vi "GetProbePlanCoordinates.vi"(8 "Use index as X coord":bool=TRUE, 9 "Probe Card Channels":i32=1) -> (0 "file path":string="C:\\Users\\itk\\Documents\\itk-strip-sensor-qc\\ProbePlans\\190723_ATLAS18R0_layer5__ATLAS18R0_ACPads.txt", 2 "OK?":bool=TRUE, 3 "Array":T1(array[cluster])=[{"Region"="Segment\t0T", "ProbePoints"=[{"X"=1.0, "Y"=0.0, "Label"="Strip\t1", "Coord On/Off"=TRUE}, {"X"=2.0, "Y"=0.0, "Label"="Strip\t2", "Coord On/Off"=TRUE}, {"X"=3.0, "Y"=0.0, "Label"="Strip\t3", "Coord On/Off"=TRUE}, {"X"=4.0, "Y"=0.0, "Label"="Strip\t4", "Coord On/Off"=TRUE}, {"X"=5.0, "Y"=0.0, "Label"="Strip\t5", "Coord On/Off"=TRUE}, {"X"=6.0, "Y"=0.0, "Label"="Strip\t6", "Coord On/Off"=TRUE}, {"X"=7.0, "Y"=0.0, "Label"="Strip\t7", "Coord On/Off"=TRUE}, {"X"=8.0, "Y"=0.0, "Label"="Strip\t8", "Coord On/Off"=TRUE}, {"X"=9.0, "Y"=0.0, "Label"="Strip\t9", "Coord On/Off"=TRUE}, {"X"=10.0, "Y"=0.0, "Label"="Strip\t10", "Coord On/Off"=TRUE}, {"X"=11.0, "Y"=0.0, "Label"="Strip\t11", "Coord On/Off"=TRUE}, {"X"=12.0, "Y"=0.0, "Label"="Strip\t12", "Coord On/Off"=TRUE}, {"X"=13.0, "Y"=0.0, "Label"="Strip\t13", "Coord On/Off"=TRUE}, {"X"=14.0, "Y"=0.0, "Label"="Strip\t14", "Coord On/Off"=TRUE}, {"X"=15.0, "Y"=0.0, "Label"="Strip\t15", "Coord On/Off"=TRUE}, {"X"=16.0, "Y"=0.0, "Label"="Strip\t16", "Coord On/Off"=TRUE}, {"X"=17.0, "Y"=0.0, "Label"="Strip\t17", "Coord On/Off"=TRUE}, {"X"=18.0, "Y"=0.0, "Label"="Strip\t18", "Coord On/Off"=TRUE}, {"X"=19.0, "Y"=0.0, "Label"="Strip\t19", "Coord On/Off"=TRUE}, {"X"=20.0, "Y"=0.0, "Label"="Strip\t20", "Coord On/Off"=TRUE}, {"X"=21.0, "Y"=0.0, "Label"="Strip\t21", "Coord On/Off"=TRUE}, {"X"=22.0, "Y"=0.0, "Label"="Strip\t22", "Coord On/Off"=TRUE}, {"X"=23.0, "Y"=0.0, "Label"="Strip\t23", "Coord On/Off"=TRUE}, {"X"=24.0, "Y"=0.0, "Label"="Strip\t24", "Coord On/Off"=TRUE}, {"X"=25.0, "Y"=0.0, "Label"="Strip\t25", "Coord On/Off"=TRUE}, {"X"=26.0, "Y"=0.0, "Label"="Strip\t26", "Coord On/Off"=TRUE}, {"X"=27.0, "Y"=0.0, "Label"="Strip\t27", "Coord On/Off"=TRUE}, {"X"=28.0, "Y"=0.0, "Label"="Strip\t28", "Coord On/Off"=TRUE}, {"X"=29.0, "Y"=0.0, "Label"="Strip\t29", "Coord On/Off"=TRUE}, {"X"=30.0, "Y"=0.0, "Label"="Strip\t30", "Coord On/Off"=TRUE}, {"X"=31.0, "Y"=0.0, "Label"="Strip\t31", "Coord On/Off"=TRUE}, {"X"=32.0, "Y"=0.0, "Label"="Strip\t32", "Coord On/Off"=TRUE}, {"X"=33.0, "Y"=0.0, "Label"="Strip\t33", "Coord On/Off"=TRUE}, {"X"=34.0, "Y"=0.0, "Label"="Strip\t34", "Coord On/Off"=TRUE}, {"X"=35.0, "Y"=0.0, "Label"="Strip\t35", "Coord On/Off"=TRUE}, {"X"=36.0, "Y"=0.0, "Label"="Strip\t36", "Coord On/Off"=TRUE}, {"X"=37.0, "Y"=0.0, "Label"="Strip\t37", "Coord On/Off"=TRUE}, {"X"=38.0, "Y"=0.0, "Label"="Strip\t38", "Coord On/Off"=TRUE}, {"X"=39.0, "Y"=0.0, "Label"="Strip\t39", "Coord On/Off"=TRUE}, {"X"=40.0, "Y"=0.0, "Label"="Strip\t40", "Coord On/Off"=TRUE}, {"X"=41.0, "Y"=0.0, "Label"="Strip\t41", "Coord On/Off"=TRUE}, {"X"=42.0, "Y"=0.0, "Label"="Strip\t42", "Coord On/Off"=TRUE}, {"X"=43.0, "Y"=0.0, "Label"="Strip\t43", "Coord On/Off"=TRUE}, {"X"=44.0, "Y"=0.0, "Label"="Strip\t44", "Coord On/Off"=TRUE}, {"X"=45.0, "Y"=0.0, "Label"="Strip\t45", "Coord On/Off"=TRUE}, {"X"=46.0, "Y"=0.0, "Label"="Strip\t46", "Coord On/Off"=TRUE}, {"X"=47.0, "Y"=0.0, "Label"="Strip\t47", "Coord On/Off"=TRUE}, {"X"=48.0, "Y"=0.0, "Label"="Strip\t48", "Coord On/Off"=TRUE}, {"X"=49.0, "Y"=0.0, "Label"="Strip\t49", "Coord On/Off"=TRUE}, {"X"=50.0, "Y"=0.0, "Label"="Strip\t50", "Coord On/Off"=TRUE}, {"X"=51.0, "Y"=0.0, "Label"="Strip\t51", "Coord On/Off"=TRUE}, {"X"=52.0, "Y"=0.0, "Label"="Strip\t52", "Coord On/Off"=TRUE}, {"X"=53.0, "Y"=0.0, "Label"="Strip\t53", "Coord On/Off"=TRUE}, {"X"=54.0, "Y"=0.0, "Label"="Strip\t54", "Coord On/Off"=TRUE}, {"X"=55.0, "Y"=0.0, "Label"="Strip\t55", "Coord On/Off"=TRUE}, {"X"=56.0, "Y"=0.0, "Label"="Strip\t56", "Coord On/Off"=TRUE}, {"X"=57.0, "Y"=0.0, "Label"="Strip\t57", "Coord On/Off"=TRUE}, {"X"=58.0, "Y"=0.0, "Label"="Strip\t58", "Coord On/Off"=TRUE}, {"X"=59.0, "Y"=0.0, "Label"="Strip\t59", "Coord On/Off"=TRUE}, {"X"=60.0, "Y"=0.0, "Label"="Strip\t60", "Coord On/Off"=TRUE}, {"X"=61.0, "Y"=0.0, "Label"="Strip\t61", "Coord On/Off"=TRUE}, {"X"=62.0, "Y"=0.0, "Label"="Strip\t62", "Coord On/Off"=TRUE}, {"X"=63.0, "Y"=0.0, "Label"="Strip\t63", "Coord On/Off"=TRUE}, {"X"=64.0, "Y"=0.0, "Label"="Strip\t64", "Coord On/Off"=TRUE}, {"X"=65.0, "Y"=0.0, "Label"="Strip\t65", "Coord On/Off"=TRUE}, {"X"=66.0, "Y"=0.0, "Label"="Strip\t66", "Coord On/Off"=TRUE}, {"X"=67.0, "Y"=0.0, "Label"="Strip\t67", "Coord On/Off"=TRUE}, {"X"=68.0, "Y"=0.0, "Label"="Strip\t68", "Coord On/Off"=TRUE}, {"X"=69.0, "Y"=0.0, "Label"="Strip\t69", "Coord On/Off"=TRUE}, {"X"=70.0, "Y"=0.0, "Label"="Strip\t70", "Coord On/Off"=TRUE}, {"X"=71.0, "Y"=0.0, "Label"="Strip\t71", "Coord On/Off"=TRUE}, {"X"=72.0, "Y"=0.0, "Label"="Strip\t72", "Coord On/Off"=TRUE}, {"X"=73.0, "Y"=0.0, "Label"="Strip\t73", "Coord On/Off"=TRUE}, {"X"=74.0, "Y"=0.0, "Label"="Strip\t74", "Coord On/Off"=TRUE}, {"X"=75.0, "Y"=0.0, "Label"="Strip\t75", "Coord On/Off"=TRUE}, {"X"=76.0, "Y"=0.0, "Label"="Strip\t76", "Coord On/Off"=TRUE}, {"X"=77.0, "Y"=0.0, "Label"="Strip\t77", "Coord On/Off"=TRUE}, {"X"=78.0, "Y"=0.0, "Label"="Strip\t78", "Coord On/Off"=TRUE}, {"X"=79.0, "Y"=0.0, "Label"="Strip\t79", "Coord On/Off"=TRUE}, {"X"=80.0, "Y"=0.0, "Label"="Strip\t80", "Coord On/Off"=TRUE}, {"X"=81.0, "Y"=0.0, "Label"="Strip\t81", "Coord On/Off"=TRUE}, {"X"=82.0, "Y"=0.0, "Label"="Strip\t82", "Coord On/Off"=TRUE}, {"X"=83.0, "Y"=0.0, "Label"="Strip\t83", "Coord On/Off"=TRUE}, {"X"=84.0, "Y"=0.0, "Label"="Strip\t84", "Coord On/Off"=TRUE}, {"X"=85.0, "Y"=0.0, "Label"="Strip\t85", "Coord On/Off"=TRUE}, {"X"=86.0, "Y"=0.0, "Label"="Strip\t86", "Coord On/Off"=TRUE}, {"X"=87.0, "Y"=0.0, "Label"="Strip\t87", "Coord On/Off"=TRUE}, {"X"=88.0, "Y"=0.0, "Label"="Strip\t88", "Coord On/Off"=TRUE}, {"X"=89.0, "Y"=0.0, "Label"="Strip\t89", "Coord On/Off"=TRUE}, {"X"=90.0, "Y"=0.0, "Label"="Strip\t90", "Coord On/Off"=TRUE}, {"X"=91.0, "Y"=0.0, "Label"="Strip\t91", "Coord On/Off"=TRUE}, {"X"=92.0, "Y"=0.0, "Label"="Strip\t92", "Coord On/Off"=TRUE}, {"X"=93.0, "Y"=0.0, "Label"="Strip\t93", "Coord On/Off"=TRUE}, {"X"=94.0, "Y"=0.0, "Label"="Strip\t94", "Coord On/Off"=TRUE}, {"X"=95.0, "Y"=0.0, "Label"="Strip\t95", "Coord On/Off"=TRUE}, {"X"=96.0, "Y"=0.0, "Label"="Strip\t96", "Coord On/Off"=TRUE}, {"X"=97.0, "Y"=0.0, "Label"="Strip\t97", "Coord On/Off"=TRUE}, {"X"=98.0, "Y"=0.0, "Label"="Strip\t98", "Coord On/Off"=TRUE}, {"X"=99.0, "Y"=0.0, "Label"="Strip\t99", "Coord On/Off"=TRUE}, {"X"=100.0, "Y"=0.0, "Label"="Strip\t100", "Coord On/Off"=TRUE}, {"X"=101.0, "Y"=0.0, "Label"="Strip\t101", "Coord On/Off"=TRUE}, {"X"=102.0, "Y"=0.0, "Label"="Strip\t102", "Coord On/Off"=TRUE}, {"X"=103.0, "Y"=0.0, "Label"="Strip\t103", "Coord On/Off"=TRUE}, {"X"=104.0, "Y"=0.0, "Label"="Strip\t104", "Coord On/Off"=TRUE}, {"X"=105.0, "Y"=0.0, "Label"="Strip\t105", "Coord On/Off"=TRUE}, {"X"=106.0, "Y"=0.0, "Label"="Strip\t106", "Coord On/Off"=TRUE}, {"X"=107.0, "Y"=0.0, "Label"="Strip\t107", "Coord On/Off"=TRUE}, {"X"=108.0, "Y"=0.0, "Label"="Strip\t108", "Coord On/Off"=TRUE}, {"X"=109.0, "Y"=0.0, "Label"="Strip\t109", "Coord On/Off"=TRUE}, {"X"=110.0, "Y"=0.0, "Label"="Strip\t110", "Coord On/Off"=TRUE}, {"X"=111.0, "Y"=0.0, "Label"="Strip\t111", "Coord On/Off"=TRUE}, {"X"=112.0, "Y"=0.0, "Label"="Strip\t112", "Coord On/Off"=TRUE}, {"X"=113.0, "Y"=0.0, "Label"="Strip\t113", "Coord On/Off"=TRUE}, {"X"=114.0, "Y"=0.0, "Label"="Strip\t114", "Coord On/Off"=TRUE}, {"X"=115.0, "Y"=0.0, "Label"="Strip\t115", "Coord On/Off"=TRUE}, {"X"=116.0, "Y"=0.0, "Label"="Strip\t116", "Coord On/Off"=TRUE}, {"X"=117.0, "Y"=0.0, "Label"="Strip\t117", "Coord On/Off"=TRUE}, {"X"=118.0, "Y"=0.0, "Label"="Strip\t118", "Coord On/Off"=TRUE}, {"X"=119.0, "Y"=0.0, "Label"="Strip\t119", "Coord On/Off"=TRUE}, {"X"=120.0, "Y"=0.0, "Label"="Strip\t120", "Coord On/Off"=TRUE}, {"X"=121.0, "Y"=0.0, "Label"="Strip\t121", "Coord On/Off"=TRUE}, {"X"=122.0, "Y"=0.0, "Label"="Strip\t122", "Coord On/Off"=TRUE}, {"X"=123.0, "Y"=0.0, "Label"="Strip\t123", "Coord On/Off"=TRUE}, {"X"=124.0, "Y"=0.0, "Label"="Strip\t124", "Coord On/Off"=TRUE}, {"X"=125.0, "Y"=0.0, "Label"="Strip\t125", "Coord On/Off"=TRUE}, {"X"=126.0, "Y"=0.0, "Label"="Strip\t126", "Coord On/Off"=TRUE}, {"X"=127.0, "Y"=0.0, "Label"="Strip\t127", "Coord On/Off"=TRUE}, {"X"=128.0, "Y"=0.0, "Label"="Strip\t128", "Coord On/Off"=TRUE}, {"X"=129.0, "Y"=0.0, "Label"="Strip\t129", "Coord On/Off"=TRUE}, {"X"=130.0, "Y"=0.0, "Label"="Strip\t130", "Coord On/Off"=TRUE}, {"X"=131.0, "Y"=0.0, "Label"="Strip\t131", "Coord On/Off"=TRUE}, {"X"=132.0, "Y"=0.0, "Label"="Strip\t132", "Coord On/Off"=TRUE}, {"X"=133.0, "Y"=0.0, "Label"="Strip\t133", "Coord On/Off"=TRUE}, {"X"=134.0, "Y"=0.0, "Label"="Strip\t134", "Coord On/Off"=TRUE}, {"X"=135.0, "Y"=0.0, "Label"="Strip\t135", "Coord On/Off"=TRUE}, {"X"=136.0, "Y"=0.0, "Label"="Strip\t136", "Coord On/Off"=TRUE}, {"X"=137.0, "Y"=0.0, "Label"="Strip\t137", "Coord On/Off"=TRUE}, {"X"=138.0, "Y"=0.0, "Label"="Strip\t138", "Coord On/Off"=TRUE}, {"X"=139.0, "Y"=0.0, "Label"="Strip\t139", "Coord On/Off"=TRUE}, {"X"=140.0, "Y"=0.0, "Label"="Strip\t140", "Coord On/Off"=TRUE}, {"X"=141.0, "Y"=0.0, "Label"="Strip\t141", "Coord On/Off"=TRUE}, {"X"=142.0, "Y"=0.0, "Label"="Strip\t142", "Coord On/Off"=TRUE}, {"X"=143.0, "Y"=0.0, "Label"="Strip\t143", "Coord On/Off"=TRUE}, {"X"=144.0, "Y"=0.0, "Label"="Strip\t144", "Coord On/Off"=TRUE}, {"X"=145.0, "Y"=0.0, "Label"="Strip\t145", "Coord On/Off"=TRUE}, {"X"=146.0, "Y"=0.0, "Label"="Strip\t146", "Coord On/Off"=TRUE}, {"X"=147.0, "Y"=0.0, "Label"="Strip\t147", "Coord On/Off"=TRUE}, {"X"=148.0, "Y"=0.0, "Label"="Strip\t148", "Coord On/Off"=TRUE}, {"X"=149.0, "Y"=0.0, "Label"="Strip\t149", "Coord On/Off"=TRUE}, {"X"=150.0, "Y"=0.0, "Label"="Strip\t150", "Coord On/Off"=TRUE}, {"X"=151.0, "Y"=0.0, "Label"="Strip\t151", "Coord On/Off"=TRUE}, {"X"=152.0, "Y"=0.0, "Label"="Strip\t152", "Coord On/Off"=TRUE}, {"X"=153.0, "Y"=0.0, "Label"="Strip\t153", "Coord On/Off"=TRUE}, {"X"=154.0, "Y"=0.0, "Label"="Strip\t154", "Coord On/Off"=TRUE}, {"X"=155.0, "Y"=0.0, "Label"="Strip\t155", "Coord On/Off"=TRUE}, {"X"=156.0, "Y"=0.0, "Label"="Strip\t156", "Coord On/Off"=TRUE}, {"X"=157.0, "Y"=0.0, "Label"="Strip\t157", "Coord On/Off"=TRUE}, {"X"=158.0, "Y"=0.0, "Label"="Strip\t158", "Coord On/Off"=TRUE}, {"X"=159.0, "Y"=0.0, "Label"="Strip\t159", "Coord On/Off"=TRUE}, {"X"=160.0, "Y"=0.0, "Label"="Strip\t160", "Coord On/Off"=TRUE}, {"X"=161.0, "Y"=0.0, "Label"="Strip\t161", "Coord On/Off"=TRUE}, {"X"=162.0, "Y"=0.0, "Label"="Strip\t162", "Coord On/Off"=TRUE}, {"X"=163.0, "Y"=0.0, "Label"="Strip\t163", "Coord On/Off"=TRUE}, {"X"=164.0, "Y"=0.0, "Label"="Strip\t164", "Coord On/Off"=TRUE}, {"X"=165.0, "Y"=0.0, "Label"="Strip\t165", "Coord On/Off"=TRUE}, {"X"=166.0, "Y"=0.0, "Label"="Strip\t166", "Coord On/Off"=TRUE}, {"X"=167.0, "Y"=0.0, "Label"="Strip\t167", "Coord On/Off"=TRUE}, {"X"=168.0, "Y"=0.0, "Label"="Strip\t168", "Coord On/Off"=TRUE}, {"X"=169.0, "Y"=0.0, "Label"="Strip\t169", "Coord On/Off"=TRUE}, {"X"=170.0, "Y"=0.0, "Label"="Strip\t170", "Coord On/Off"=TRUE}, {"X"=171.0, "Y"=0.0, "Label"="Strip\t171", "Coord On/Off"=TRUE}, {"X"=172.0, "Y"=0.0, "Label"="Strip\t172", "Coord On/Off"=TRUE}, {"X"=173.0, "Y"=0.0, "Label"="Strip\t173", "Coord On/Off"=TRUE}, {"X"=174.0, "Y"=0.0, "Label"="Strip\t174", "Coord On/Off"=TRUE}, {"X"=175.0, "Y"=0.0, "Label"="Strip\t175", "Coord On/Off"=TRUE}, {"X"=176.0, "Y"=0.0, "Label"="Strip\t176", "Coord On/Off"=TRUE}, {"X"=177.0, "Y"=0.0, "Label"="Strip\t177", "Coord On/Off"=TRUE}, {"X"=178.0, "Y"=0.0, "Label"="Strip\t178", "Coord On/Off"=TRUE}, {"X"=179.0, "Y"=0.0, "Label"="Strip\t179", "Coord On/Off"=TRUE}, {"X"=180.0, "Y"=0.0, "Label"="Strip\t180", "Coord On/Off"=TRUE}, {"X"=181.0, "Y"=0.0, "Label"="Strip\t181", "Coord On/Off"=TRUE}, {"X"=182.0, "Y"=0.0, "Label"="Strip\t182", "Coord On/Off"=TRUE}, {"X"=183.0, "Y"=0.0, "Label"="Strip\t183", "Coord On/Off"=TRUE}, {"X"=184.0, "Y"=0.0, "Label"="Strip\t184", "Coord On/Off"=TRUE}, {"X"=185.0, "Y"=0.0, "Label"="Strip\t185", "Coord On/Off"=TRUE}, {"X"=186.0, "Y"=0.0, "Label"="Strip\t186", "Coord On/Off"=TRUE}, {"X"=187.0, "Y"=0.0, "Label"="Strip\t187", "Coord On/Off"=TRUE}, {"X"=188.0, "Y"=0.0, "Label"="Strip\t188", "Coord On/Off"=TRUE}, {"X"=189.0, "Y"=0.0, "Label"="Strip\t189", "Coord On/Off"=TRUE}, {"X"=190.0, "Y"=0.0, "Label"="Strip\t190", "Coord On/Off"=TRUE}, {"X"=191.0, "Y"=0.0, "Label"="Strip\t191", "Coord On/Off"=TRUE}, {"X"=192.0, "Y"=0.0, "Label"="Strip\t192", "Coord On/Off"=TRUE}, {"X"=193.0, "Y"=0.0, "Label"="Strip\t193", "Coord On/Off"=TRUE}, {"X"=194.0, "Y"=0.0, "Label"="Strip\t194", "Coord On/Off"=TRUE}, {"X"=195.0, "Y"=0.0, "Label"="Strip\t195", "Coord On/Off"=TRUE}, {"X"=196.0, "Y"=0.0, "Label"="Strip\t196", "Coord On/Off"=TRUE}, {"X"=197.0, "Y"=0.0, "Label"="Strip\t197", "Coord On/Off"=TRUE}, {"X"=198.0, "Y"=0.0, "Label"="Strip\t198", "Coord On/Off"=TRUE}, {"X"=199.0, "Y"=0.0, "Label"="Strip\t199", "Coord On/Off"=TRUE}, {"X"=200.0, "Y"=0.0, "Label"="Strip\t200", "Coord On/Off"=TRUE}, {"X"=201.0, "Y"=0.0, "Label"="Strip\t201", "Coord On/Off"=TRUE}, {"X"=202.0, "Y"=0.0, "Label"="Strip\t202", "Coord On/Off"=TRUE}, {"X"=203.0, "Y"=0.0, "Label"="Strip\t203", "Coord On/Off"=TRUE}, {"X"=204.0, "Y"=0.0, "Label"="Strip\t204", "Coord On/Off"=TRUE}, {"X"=205.0, "Y"=0.0, "Label"="Strip\t205", "Coord On/Off"=TRUE}, {"X"=206.0, "Y"=0.0, "Label"="Strip\t206", "Coord On/Off"=TRUE}, {"X"=207.0, "Y"=0.0, "Label"="Strip\t207", "Coord On/Off"=TRUE}, {"X"=208.0, "Y"=0.0, "Label"="Strip\t208", "Coord On/Off"=TRUE}, {"X"=209.0, "Y"=0.0, "Label"="Strip\t209", "Coord On/Off"=TRUE}, {"X"=210.0, "Y"=0.0, "Label"="Strip\t210", "Coord On/Off"=TRUE}, {"X"=211.0, "Y"=0.0, "Label"="Strip\t211", "Coord On/Off"=TRUE}, {"X"=212.0, "Y"=0.0, "Label"="Strip\t212", "Coord On/Off"=TRUE}, {"X"=213.0, "Y"=0.0, "Label"="Strip\t213", "Coord On/Off"=TRUE}, {"X"=214.0, "Y"=0.0, "Label"="Strip\t214", "Coord On/Off"=TRUE}, {"X"=215.0, "Y"=0.0, "Label"="Strip\t215", "Coord On/Off"=TRUE}, {"X"=216.0, "Y"=0.0, "Label"="Strip\t216", "Coord On/Off"=TRUE}, {"X"=217.0, "Y"=0.0, "Label"="Strip\t217", "Coord On/Off"=TRUE}, {"X"=218.0, "Y"=0.0, "Label"="Strip\t218", "Coord On/Off"=TRUE}, {"X"=219.0, "Y"=0.0, "Label"="Strip\t219", "Coord On/Off"=TRUE}, {"X"=220.0, "Y"=0.0, "Label"="Strip\t220", "Coord On/Off"=TRUE}, {"X"=221.0, "Y"=0.0, "Label"="Strip\t221", "Coord On/Off"=TRUE}, {"X"=222.0, "Y"=0.0, "Label"="Strip\t222", "Coord On/Off"=TRUE}, {"X"=223.0, "Y"=0.0, "Label"="Strip\t223", "Coord On/Off"=TRUE}, {"X"=224.0, "Y"=0.0, "Label"="Strip\t224", "Coord On/Off"=TRUE}, {"X"=225.0, "Y"=0.0, "Label"="Strip\t225", "Coord On/Off"=TRUE}, {"X"=226.0, "Y"=0.0, "Label"="Strip\t226", "Coord On/Off"=TRUE}, {"X"=227.0, "Y"=0.0, "Label"="Strip\t227", "Coord On/Off"=TRUE}, {"X"=228.0, "Y"=0.0, "Label"="Strip\t228", "Coord On/Off"=TRUE}, {"X"=229.0, "Y"=0.0, "Label"="Strip\t229", "Coord On/Off"=TRUE}, {"X"=230.0, "Y"=0.0, "Label"="Strip\t230", "Coord On/Off"=TRUE}, {"X"=231.0, "Y"=0.0, "Label"="Strip\t231", "Coord On/Off"=TRUE}, {"X"=232.0, "Y"=0.0, "Label"="Strip\t232", "Coord On/Off"=TRUE}, {"X"=233.0, "Y"=0.0, "Label"="Strip\t233", "Coord On/Off"=TRUE}, {"X"=234.0, "Y"=0.0, "Label"="Strip\t234", "Coord On/Off"=TRUE}, {"X"=235.0, "Y"=0.0, "Label"="Strip\t235", "Coord On/Off"=TRUE}, {"X"=236.0, "Y"=0.0, "Label"="Strip\t236", "Coord On/Off"=TRUE}, {"X"=237.0, "Y"=0.0, "Label"="Strip\t237", "Coord On/Off"=TRUE}, {"X"=238.0, "Y"=0.0, "Label"="Strip\t238", "Coord On/Off"=TRUE}, {"X"=239.0, "Y"=0.0, "Label"="Strip\t239", "Coord On/Off"=TRUE}, {"X"=240.0, "Y"=0.0, "Label"="Strip\t240", "Coord On/Off"=TRUE}, {"X"=241.0, "Y"=0.0, "Label"="Strip\t241", "Coord On/Off"=TRUE}, {"X"=242.0, "Y"=0.0, "Label"="Strip\t242", "Coord On/Off"=TRUE}, {"X"=243.0, "Y"=0.0, "Label"="Strip\t243", "Coord On/Off"=TRUE}, {"X"=244.0, "Y"=0.0, "Label"="Strip\t244", "Coord On/Off"=TRUE}, {"X"=245.0, "Y"=0.0, "Label"="Strip\t245", "Coord On/Off"=TRUE}, {"X"=246.0, "Y"=0.0, "Label"="Strip\t246", "Coord On/Off"=TRUE}, {"X"=247.0, "Y"=0.0, "Label"="Strip\t247", "Coord On/Off"=TRUE}, {"X"=248.0, "Y"=0.0, "Label"="Strip\t248", "Coord On/Off"=TRUE}, {"X"=249.0, "Y"=0.0, "Label"="Strip\t249", "Coord On/Off"=TRUE}, {"X"=250.0, "Y"=0.0, "Label"="Strip\t250", "Coord On/Off"=TRUE}, {"X"=251.0, "Y"=0.0, "Label"="Strip\t251", "Coord On/Off"=TRUE}, {"X"=252.0, "Y"=0.0, "Label"="Strip\t252", "Coord On/Off"=TRUE}, {"X"=253.0, "Y"=0.0, "Label"="Strip\t253", "Coord On/Off"=TRUE}, {"X"=254.0, "Y"=0.0, "Label"="Strip\t254", "Coord On/Off"=TRUE}, {"X"=255.0, "Y"=0.0, "Label"="Strip\t255", "Coord On/Off"=TRUE}, {"X"=256.0, "Y"=0.0, "Label"="Strip\t256", "Coord On/Off"=TRUE}, {"X"=257.0, "Y"=0.0, "Label"="Strip\t257", "Coord On/Off"=TRUE}, {"X"=258.0, "Y"=0.0, "Label"="Strip\t258", "Coord On/Off"=TRUE}, {"X"=259.0, "Y"=0.0, "Label"="Strip\t259", "Coord On/Off"=TRUE}, {"X"=260.0, "Y"=0.0, "Label"="Strip\t260", "Coord On/Off"=TRUE}, {"X"=261.0, "Y"=0.0, "Label"="Strip\t261", "Coord On/Off"=TRUE}, {"X"=262.0, "Y"=0.0, "Label"="Strip\t262", "Coord On/Off"=TRUE}, {"X"=263.0, "Y"=0.0, "Label"="Strip\t263", "Coord On/Off"=TRUE}, {"X"=264.0, "Y"=0.0, "Label"="Strip\t264", "Coord On/Off"=TRUE}, {"X"=265.0, "Y"=0.0, "Label"="Strip\t265", "Coord On/Off"=TRUE}, {"X"=266.0, "Y"=0.0, "Label"="Strip\t266", "Coord On/Off"=TRUE}, {"X"=267.0, "Y"=0.0, "Label"="Strip\t267", "Coord On/Off"=TRUE}, {"X"=268.0, "Y"=0.0, "Label"="Strip\t268", "Coord On/Off"=TRUE}, {"X"=269.0, "Y"=0.0, "Label"="Strip\t269", "Coord On/Off"=TRUE}, {"X"=270.0, "Y"=0.0, "Label"="Strip\t270", "Coord On/Off"=TRUE}, {"X"=271.0, "Y"=0.0, "Label"="Strip\t271", "Coord On/Off"=TRUE}, {"X"=272.0, "Y"=0.0, "Label"="Strip\t272", "Coord On/Off"=TRUE}, {"X"=273.0, "Y"=0.0, "Label"="Strip\t273", "Coord On/Off"=TRUE}, {"X"=274.0, "Y"=0.0, "Label"="Strip\t274", "Coord On/Off"=TRUE}, {"X"=275.0, "Y"=0.0, "Label"="Strip\t275", "Coord On/Off"=TRUE}, {"X"=276.0, "Y"=0.0, "Label"="Strip\t276", "Coord On/Off"=TRUE}, {"X"=277.0, "Y"=0.0, "Label"="Strip\t277", "Coord On/Off"=TRUE}, {"X"=278.0, "Y"=0.0, "Label"="Strip\t278", "Coord On/Off"=TRUE}, {"X"=279.0, "Y"=0.0, "Label"="Strip\t279", "Coord On/Off"=TRUE}, {"X"=280.0, "Y"=0.0, "Label"="Strip\t280", "Coord On/Off"=TRUE}, {"X"=281.0, "Y"=0.0, "Label"="Strip\t281", "Coord On/Off"=TRUE}, {"X"=282.0, "Y"=0.0, "Label"="Strip\t282", "Coord On/Off"=TRUE}, {"X"=283.0, "Y"=0.0, "Label"="Strip\t283", "Coord On/Off"=TRUE}, {"X"=284.0, "Y"=0.0, "Label"="Strip\t284", "Coord On/Off"=TRUE}, {"X"=285.0, "Y"=0.0, "Label"="Strip\t285", "Coord On/Off"=TRUE}, {"X"=286.0, "Y"=0.0, "Label"="Strip\t286", "Coord On/Off"=TRUE}, {"X"=287.0, "Y"=0.0, "Label"="Strip\t287", "Coord On/Off"=TRUE}, {"X"=288.0, "Y"=0.0, "Label"="Strip\t288", "Coord On/Off"=TRUE}, {"X"=289.0, "Y"=0.0, "Label"="Strip\t289", "Coord On/Off"=TRUE}, {"X"=290.0, "Y"=0.0, "Label"="Strip\t290", "Coord On/Off"=TRUE}, {"X"=291.0, "Y"=0.0, "Label"="Strip\t291", "Coord On/Off"=TRUE}, {"X"=292.0, "Y"=0.0, "Label"="Strip\t292", "Coord On/Off"=TRUE}, {"X"=293.0, "Y"=0.0, "Label"="Strip\t293", "Coord On/Off"=TRUE}, {"X"=294.0, "Y"=0.0, "Label"="Strip\t294", "Coord On/Off"=TRUE}, {"X"=295.0, "Y"=0.0, "Label"="Strip\t295", "Coord On/Off"=TRUE}, {"X"=296.0, "Y"=0.0, "Label"="Strip\t296", "Coord On/Off"=TRUE}, {"X"=297.0, "Y"=0.0, "Label"="Strip\t297", "Coord On/Off"=TRUE}, {"X"=298.0, "Y"=0.0, "Label"="Strip\t298", "Coord On/Off"=TRUE}, {"X"=299.0, "Y"=0.0, "Label"="Strip\t299", "Coord On/Off"=TRUE}, {"X"=300.0, "Y"=0.0, "Label"="Strip\t300", "Coord On/Off"=TRUE}, {"X"=301.0, "Y"=0.0, "Label"="Strip\t301", "Coord On/Off"=TRUE}, {"X"=302.0, "Y"=0.0, "Label"="Strip\t302", "Coord On/Off"=TRUE}, {"X"=303.0, "Y"=0.0, "Label"="Strip\t303", "Coord On/Off"=TRUE}, {"X"=304.0, "Y"=0.0, "Label"="Strip\t304", "Coord On/Off"=TRUE}, {"X"=305.0, "Y"=0.0, "Label"="Strip\t305", "Coord On/Off"=TRUE}, {"X"=306.0, "Y"=0.0, "Label"="Strip\t306", "Coord On/Off"=TRUE}, {"X"=307.0, "Y"=0.0, "Label"="Strip\t307", "Coord On/Off"=TRUE}, {"X"=308.0, "Y"=0.0, "Label"="Strip\t308", "Coord On/Off"=TRUE}, {"X"=309.0, "Y"=0.0, "Label"="Strip\t309", "Coord On/Off"=TRUE}, {"X"=310.0, "Y"=0.0, "Label"="Strip\t310", "Coord On/Off"=TRUE}, {"X"=311.0, "Y"=0.0, "Label"="Strip\t311", "Coord On/Off"=TRUE}, {"X"=312.0, "Y"=0.0, "Label"="Strip\t312", "Coord On/Off"=TRUE}, {"X"=313.0, "Y"=0.0, "Label"="Strip\t313", "Coord On/Off"=TRUE}, {"X"=314.0, "Y"=0.0, "Label"="Strip\t314", "Coord On/Off"=TRUE}, {"X"=315.0, "Y"=0.0, "Label"="Strip\t315", "Coord On/Off"=TRUE}, {"X"=316.0, "Y"=0.0, "Label"="Strip\t316", "Coord On/Off"=TRUE}, {"X"=317.0, "Y"=0.0, "Label"="Strip\t317", "Coord On/Off"=TRUE}, {"X"=318.0, "Y"=0.0, "Label"="Strip\t318", "Coord On/Off"=TRUE}, {"X"=319.0, "Y"=0.0, "Label"="Strip\t319", "Coord On/Off"=TRUE}, {"X"=320.0, "Y"=0.0, "Label"="Strip\t320", "Coord On/Off"=TRUE}, {"X"=321.0, "Y"=0.0, "Label"="Strip\t321", "Coord On/Off"=TRUE}, {"X"=322.0, "Y"=0.0, "Label"="Strip\t322", "Coord On/Off"=TRUE}, {"X"=323.0, "Y"=0.0, "Label"="Strip\t323", "Coord On/Off"=TRUE}, {"X"=324.0, "Y"=0.0, "Label"="Strip\t324", "Coord On/Off"=TRUE}, {"X"=325.0, "Y"=0.0, "Label"="Strip\t325", "Coord On/Off"=TRUE}, {"X"=326.0, "Y"=0.0, "Label"="Strip\t326", "Coord On/Off"=TRUE}, {"X"=327.0, "Y"=0.0, "Label"="Strip\t327", "Coord On/Off"=TRUE}, {"X"=328.0, "Y"=0.0, "Label"="Strip\t328", "Coord On/Off"=TRUE}, {"X"=329.0, "Y"=0.0, "Label"="Strip\t329", "Coord On/Off"=TRUE}, {"X"=330.0, "Y"=0.0, "Label"="Strip\t330", "Coord On/Off"=TRUE}, {"X"=331.0, "Y"=0.0, "Label"="Strip\t331", "Coord On/Off"=TRUE}, {"X"=332.0, "Y"=0.0, "Label"="Strip\t332", "Coord On/Off"=TRUE}, {"X"=333.0, "Y"=0.0, "Label"="Strip\t333", "Coord On/Off"=TRUE}, {"X"=334.0, "Y"=0.0, "Label"="Strip\t334", "Coord On/Off"=TRUE}, {"X"=335.0, "Y"=0.0, "Label"="Strip\t335", "Coord On/Off"=TRUE}, {"X"=336.0, "Y"=0.0, "Label"="Strip\t336", "Coord On/Off"=TRUE}, {"X"=337.0, "Y"=0.0, "Label"="Strip\t337", "Coord On/Off"=TRUE}, {"X"=338.0, "Y"=0.0, "Label"="Strip\t338", "Coord On/Off"=TRUE}, {"X"=339.0, "Y"=0.0, "Label"="Strip\t339", "Coord On/Off"=TRUE}, {"X"=340.0, "Y"=0.0, "Label"="Strip\t340", "Coord On/Off"=TRUE}, {"X"=341.0, "Y"=0.0, "Label"="Strip\t341", "Coord On/Off"=TRUE}, {"X"=342.0, "Y"=0.0, "Label"="Strip\t342", "Coord On/Off"=TRUE}, {"X"=343.0, "Y"=0.0, "Label"="Strip\t343", "Coord On/Off"=TRUE}, {"X"=344.0, "Y"=0.0, "Label"="Strip\t344", "Coord On/Off"=TRUE}, {"X"=345.0, "Y"=0.0, "Label"="Strip\t345", "Coord On/Off"=TRUE}, {"X"=346.0, "Y"=0.0, "Label"="Strip\t346", "Coord On/Off"=TRUE}, {"X"=347.0, "Y"=0.0, "Label"="Strip\t347", "Coord On/Off"=TRUE}, {"X"=348.0, "Y"=0.0, "Label"="Strip\t348", "Coord On/Off"=TRUE}, {"X"=349.0, "Y"=0.0, "Label"="Strip\t349", "Coord On/Off"=TRUE}, {"X"=350.0, "Y"=0.0, "Label"="Strip\t350", "Coord On/Off"=TRUE}, {"X"=351.0, "Y"=0.0, "Label"="Strip\t351", "Coord On/Off"=TRUE}, {"X"=352.0, "Y"=0.0, "Label"="Strip\t352", "Coord On/Off"=TRUE}, {"X"=353.0, "Y"=0.0, "Label"="Strip\t353", "Coord On/Off"=TRUE}, {"X"=354.0, "Y"=0.0, "Label"="Strip\t354", "Coord On/Off"=TRUE}, {"X"=355.0, "Y"=0.0, "Label"="Strip\t355", "Coord On/Off"=TRUE}, {"X"=356.0, "Y"=0.0, "Label"="Strip\t356", "Coord On/Off"=TRUE}, {"X"=357.0, "Y"=0.0, "Label"="Strip\t357", "Coord On/Off"=TRUE}, {"X"=358.0, "Y"=0.0, "Label"="Strip\t358", "Coord On/Off"=TRUE}, {"X"=359.0, "Y"=0.0, "Label"="Strip\t359", "Coord On/Off"=TRUE}, {"X"=360.0, "Y"=0.0, "Label"="Strip\t360", "Coord On/Off"=TRUE}, {"X"=361.0, "Y"=0.0, "Label"="Strip\t361", "Coord On/Off"=TRUE}, {"X"=362.0, "Y"=0.0, "Label"="Strip\t362", "Coord On/Off"=TRUE}, {"X"=363.0, "Y"=0.0, "Label"="Strip\t363", "Coord On/Off"=TRUE}, {"X"=364.0, "Y"=0.0, "Label"="Strip\t364", "Coord On/Off"=TRUE}, {"X"=365.0, "Y"=0.0, "Label"="Strip\t365", "Coord On/Off"=TRUE}, {"X"=366.0, "Y"=0.0, "Label"="Strip\t366", "Coord On/Off"=TRUE}, {"X"=367.0, "Y"=0.0, "Label"="Strip\t367", "Coord On/Off"=TRUE}, {"X"=368.0, "Y"=0.0, "Label"="Strip\t368", "Coord On/Off"=TRUE}, {"X"=369.0, "Y"=0.0, "Label"="Strip\t369", "Coord On/Off"=TRUE}, {"X"=370.0, "Y"=0.0, "Label"="Strip\t370", "Coord On/Off"=TRUE}, {"X"=371.0, "Y"=0.0, "Label"="Strip\t371", "Coord On/Off"=TRUE}, {"X"=372.0, "Y"=0.0, "Label"="Strip\t372", "Coord On/Off"=TRUE}, {"X"=373.0, "Y"=0.0, "Label"="Strip\t373", "Coord On/Off"=TRUE}, {"X"=374.0, "Y"=0.0, "Label"="Strip\t374", "Coord On/Off"=TRUE}, {"X"=375.0, "Y"=0.0, "Label"="Strip\t375", "Coord On/Off"=TRUE}, {"X"=376.0, "Y"=0.0, "Label"="Strip\t376", "Coord On/Off"=TRUE}, {"X"=377.0, "Y"=0.0, "Label"="Strip\t377", "Coord On/Off"=TRUE}, {"X"=378.0, "Y"=0.0, "Label"="Strip\t378", "Coord On/Off"=TRUE}, {"X"=379.0, "Y"=0.0, "Label"="Strip\t379", "Coord On/Off"=TRUE}, {"X"=380.0, "Y"=0.0, "Label"="Strip\t380", "Coord On/Off"=TRUE}, {"X"=381.0, "Y"=0.0, "Label"="Strip\t381", "Coord On/Off"=TRUE}, {"X"=382.0, "Y"=0.0, "Label"="Strip\t382", "Coord On/Off"=TRUE}, {"X"=383.0, "Y"=0.0, "Label"="Strip\t383", "Coord On/Off"=TRUE}, {"X"=384.0, "Y"=0.0, "Label"="Strip\t384", "Coord On/Off"=TRUE}, {"X"=385.0, "Y"=0.0, "Label"="Strip\t385", "Coord On/Off"=TRUE}, {"X"=386.0, "Y"=0.0, "Label"="Strip\t386", "Coord On/Off"=TRUE}, {"X"=387.0, "Y"=0.0, "Label"="Strip\t387", "Coord On/Off"=TRUE}, {"X"=388.0, "Y"=0.0, "Label"="Strip\t388", "Coord On/Off"=TRUE}, {"X"=389.0, "Y"=0.0, "Label"="Strip\t389", "Coord On/Off"=TRUE}, {"X"=390.0, "Y"=0.0, "Label"="Strip\t390", "Coord On/Off"=TRUE}, {"X"=391.0, "Y"=0.0, "Label"="Strip\t391", "Coord On/Off"=TRUE}, {"X"=392.0, "Y"=0.0, "Label"="Strip\t392", "Coord On/Off"=TRUE}, {"X"=393.0, "Y"=0.0, "Label"="Strip\t393", "Coord On/Off"=TRUE}, {"X"=394.0, "Y"=0.0, "Label"="Strip\t394", "Coord On/Off"=TRUE}, {"X"=395.0, "Y"=0.0, "Label"="Strip\t395", "Coord On/Off"=TRUE}, {"X"=396.0, "Y"=0.0, "Label"="Strip\t396", "Coord On/Off"=TRUE}, {"X"=397.0, "Y"=0.0, "Label"="Strip\t397", "Coord On/Off"=TRUE}, {"X"=398.0, "Y"=0.0, "Label"="Strip\t398", "Coord On/Off"=TRUE}, {"X"=399.0, "Y"=0.0, "Label"="Strip\t399", "Coord On/Off"=TRUE}, {"X"=400.0, "Y"=0.0, "Label"="Strip\t400", "Coord On/Off"=TRUE}, {"X"=401.0, "Y"=0.0, "Label"="Strip\t401", "Coord On/Off"=TRUE}, {"X"=402.0, "Y"=0.0, "Label"="Strip\t402", "Coord On/Off"=TRUE}, {"X"=403.0, "Y"=0.0, "Label"="Strip\t403", "Coord On/Off"=TRUE}, {"X"=404.0, "Y"=0.0, "Label"="Strip\t404", "Coord On/Off"=TRUE}, {"X"=405.0, "Y"=0.0, "Label"="Strip\t405", "Coord On/Off"=TRUE}, {"X"=406.0, "Y"=0.0, "Label"="Strip\t406", "Coord On/Off"=TRUE}, {"X"=407.0, "Y"=0.0, "Label"="Strip\t407", "Coord On/Off"=TRUE}, {"X"=408.0, "Y"=0.0, "Label"="Strip\t408", "Coord On/Off"=TRUE}, {"X"=409.0, "Y"=0.0, "Label"="Strip\t409", "Coord On/Off"=TRUE}, {"X"=410.0, "Y"=0.0, "Label"="Strip\t410", "Coord On/Off"=TRUE}, {"X"=411.0, "Y"=0.0, "Label"="Strip\t411", "Coord On/Off"=TRUE}, {"X"=412.0, "Y"=0.0, "Label"="Strip\t412", "Coord On/Off"=TRUE}, {"X"=413.0, "Y"=0.0, "Label"="Strip\t413", "Coord On/Off"=TRUE}, {"X"=414.0, "Y"=0.0, "Label"="Strip\t414", "Coord On/Off"=TRUE}, {"X"=415.0, "Y"=0.0, "Label"="Strip\t415", "Coord On/Off"=TRUE}, {"X"=416.0, "Y"=0.0, "Label"="Strip\t416", "Coord On/Off"=TRUE}, {"X"=417.0, "Y"=0.0, "Label"="Strip\t417", "Coord On/Off"=TRUE}, {"X"=418.0, "Y"=0.0, "Label"="Strip\t418", "Coord On/Off"=TRUE}, {"X"=419.0, "Y"=0.0, "Label"="Strip\t419", "Coord On/Off"=TRUE}, {"X"=420.0, "Y"=0.0, "Label"="Strip\t420", "Coord On/Off"=TRUE}, {"X"=421.0, "Y"=0.0, "Label"="Strip\t421", "Coord On/Off"=TRUE}, {"X"=422.0, "Y"=0.0, "Label"="Strip\t422", "Coord On/Off"=TRUE}, {"X"=423.0, "Y"=0.0, "Label"="Strip\t423", "Coord On/Off"=TRUE}, {"X"=424.0, "Y"=0.0, "Label"="Strip\t424", "Coord On/Off"=TRUE}, {"X"=425.0, "Y"=0.0, "Label"="Strip\t425", "Coord On/Off"=TRUE}, {"X"=426.0, "Y"=0.0, "Label"="Strip\t426", "Coord On/Off"=TRUE}, {"X"=427.0, "Y"=0.0, "Label"="Strip\t427", "Coord On/Off"=TRUE}, {"X"=428.0, "Y"=0.0, "Label"="Strip\t428", "Coord On/Off"=TRUE}, {"X"=429.0, "Y"=0.0, "Label"="Strip\t429", "Coord On/Off"=TRUE}, {"X"=430.0, "Y"=0.0, "Label"="Strip\t430", "Coord On/Off"=TRUE}, {"X"=431.0, "Y"=0.0, "Label"="Strip\t431", "Coord On/Off"=TRUE}, {"X"=432.0, "Y"=0.0, "Label"="Strip\t432", "Coord On/Off"=TRUE}, {"X"=433.0, "Y"=0.0, "Label"="Strip\t433", "Coord On/Off"=TRUE}, {"X"=434.0, "Y"=0.0, "Label"="Strip\t434", "Coord On/Off"=TRUE}, {"X"=435.0, "Y"=0.0, "Label"="Strip\t435", "Coord On/Off"=TRUE}, {"X"=436.0, "Y"=0.0, "Label"="Strip\t436", "Coord On/Off"=TRUE}, {"X"=437.0, "Y"=0.0, "Label"="Strip\t437", "Coord On/Off"=TRUE}, {"X"=438.0, "Y"=0.0, "Label"="Strip\t438", "Coord On/Off"=TRUE}, {"X"=439.0, "Y"=0.0, "Label"="Strip\t439", "Coord On/Off"=TRUE}, {"X"=440.0, "Y"=0.0, "Label"="Strip\t440", "Coord On/Off"=TRUE}, {"X"=441.0, "Y"=0.0, "Label"="Strip\t441", "Coord On/Off"=TRUE}, {"X"=442.0, "Y"=0.0, "Label"="Strip\t442", "Coord On/Off"=TRUE}, {"X"=443.0, "Y"=0.0, "Label"="Strip\t443", "Coord On/Off"=TRUE}, {"X"=444.0, "Y"=0.0, "Label"="Strip\t444", "Coord On/Off"=TRUE}, {"X"=445.0, "Y"=0.0, "Label"="Strip\t445", "Coord On/Off"=TRUE}, {"X"=446.0, "Y"=0.0, "Label"="Strip\t446", "Coord On/Off"=TRUE}, {"X"=447.0, "Y"=0.0, "Label"="Strip\t447", "Coord On/Off"=TRUE}, {"X"=448.0, "Y"=0.0, "Label"="Strip\t448", "Coord On/Off"=TRUE}, {"X"=449.0, "Y"=0.0, "Label"="Strip\t449", "Coord On/Off"=TRUE}, {"X"=450.0, "Y"=0.0, "Label"="Strip\t450", "Coord On/Off"=TRUE}, {"X"=451.0, "Y"=0.0, "Label"="Strip\t451", "Coord On/Off"=TRUE}, {"X"=452.0, "Y"=0.0, "Label"="Strip\t452", "Coord On/Off"=TRUE}, {"X"=453.0, "Y"=0.0, "Label"="Strip\t453", "Coord On/Off"=TRUE}, {"X"=454.0, "Y"=0.0, "Label"="Strip\t454", "Coord On/Off"=TRUE}, {"X"=455.0, "Y"=0.0, "Label"="Strip\t455", "Coord On/Off"=TRUE}, {"X"=456.0, "Y"=0.0, "Label"="Strip\t456", "Coord On/Off"=TRUE}, {"X"=457.0, "Y"=0.0, "Label"="Strip\t457", "Coord On/Off"=TRUE}, {"X"=458.0, "Y"=0.0, "Label"="Strip\t458", "Coord On/Off"=TRUE}, {"X"=459.0, "Y"=0.0, "Label"="Strip\t459", "Coord On/Off"=TRUE}, {"X"=460.0, "Y"=0.0, "Label"="Strip\t460", "Coord On/Off"=TRUE}, {"X"=461.0, "Y"=0.0, "Label"="Strip\t461", "Coord On/Off"=TRUE}, {"X"=462.0, "Y"=0.0, "Label"="Strip\t462", "Coord On/Off"=TRUE}, {"X"=463.0, "Y"=0.0, "Label"="Strip\t463", "Coord On/Off"=TRUE}, {"X"=464.0, "Y"=0.0, "Label"="Strip\t464", "Coord On/Off"=TRUE}, {"X"=465.0, "Y"=0.0, "Label"="Strip\t465", "Coord On/Off"=TRUE}, {"X"=466.0, "Y"=0.0, "Label"="Strip\t466", "Coord On/Off"=TRUE}, {"X"=467.0, "Y"=0.0, "Label"="Strip\t467", "Coord On/Off"=TRUE}, {"X"=468.0, "Y"=0.0, "Label"="Strip\t468", "Coord On/Off"=TRUE}, {"X"=469.0, "Y"=0.0, "Label"="Strip\t469", "Coord On/Off"=TRUE}, {"X"=470.0, "Y"=0.0, "Label"="Strip\t470", "Coord On/Off"=TRUE}, {"X"=471.0, "Y"=0.0, "Label"="Strip\t471", "Coord On/Off"=TRUE}, {"X"=472.0, "Y"=0.0, "Label"="Strip\t472", "Coord On/Off"=TRUE}, {"X"=473.0, "Y"=0.0, "Label"="Strip\t473", "Coord On/Off"=TRUE}, {"X"=474.0, "Y"=0.0, "Label"="Strip\t474", "Coord On/Off"=TRUE}, {"X"=475.0, "Y"=0.0, "Label"="Strip\t475", "Coord On/Off"=TRUE}, {"X"=476.0, "Y"=0.0, "Label"="Strip\t476", "Coord On/Off"=TRUE}, {"X"=477.0, "Y"=0.0, "Label"="Strip\t477", "Coord On/Off"=TRUE}, {"X"=478.0, "Y"=0.0, "Label"="Strip\t478", "Coord On/Off"=TRUE}, {"X"=479.0, "Y"=0.0, "Label"="Strip\t479", "Coord On/Off"=TRUE}, {"X"=480.0, "Y"=0.0, "Label"="Strip\t480", "Coord On/Off"=TRUE}, {"X"=481.0, "Y"=0.0, "Label"="Strip\t481", "Coord On/Off"=TRUE}, {"X"=482.0, "Y"=0.0, "Label"="Strip\t482", "Coord On/Off"=TRUE}, {"X"=483.0, "Y"=0.0, "Label"="Strip\t483", "Coord On/Off"=TRUE}, {"X"=484.0, "Y"=0.0, "Label"="Strip\t484", "Coord On/Off"=TRUE}, {"X"=485.0, "Y"=0.0, "Label"="Strip\t485", "Coord On/Off"=TRUE}, {"X"=486.0, "Y"=0.0, "Label"="Strip\t486", "Coord On/Off"=TRUE}, {"X"=487.0, "Y"=0.0, "Label"="Strip\t487", "Coord On/Off"=TRUE}, {"X"=488.0, "Y"=0.0, "Label"="Strip\t488", "Coord On/Off"=TRUE}, {"X"=489.0, "Y"=0.0, "Label"="Strip\t489", "Coord On/Off"=TRUE}, {"X"=490.0, "Y"=0.0, "Label"="Strip\t490", "Coord On/Off"=TRUE}, {"X"=491.0, "Y"=0.0, "Label"="Strip\t491", "Coord On/Off"=TRUE}, {"X"=492.0, "Y"=0.0, "Label"="Strip\t492", "Coord On/Off"=TRUE}, {"X"=493.0, "Y"=0.0, "Label"="Strip\t493", "Coord On/Off"=TRUE}, {"X"=494.0, "Y"=0.0, "Label"="Strip\t494", "Coord On/Off"=TRUE}, {"X"=495.0, "Y"=0.0, "Label"="Strip\t495", "Coord On/Off"=TRUE}, {"X"=496.0, "Y"=0.0, "Label"="Strip\t496", "Coord On/Off"=TRUE}, {"X"=497.0, "Y"=0.0, "Label"="Strip\t497", "Coord On/Off"=TRUE}, {"X"=498.0, "Y"=0.0, "Label"="Strip\t498", "Coord On/Off"=TRUE}, {"X"=499.0, "Y"=0.0, "Label"="Strip\t499", "Coord On/Off"=TRUE}, {"X"=500.0, "Y"=0.0, "Label"="Strip\t500", "Coord On/Off"=TRUE}, {"X"=501.0, "Y"=0.0, "Label"="Strip\t501", "Coord On/Off"=TRUE}, {"X"=502.0, "Y"=0.0, "Label"="Strip\t502", "Coord On/Off"=TRUE}, {"X"=503.0, "Y"=0.0, "Label"="Strip\t503", "Coord On/Off"=TRUE}, {"X"=504.0, "Y"=0.0, "Label"="Strip\t504", "Coord On/Off"=TRUE}, {"X"=505.0, "Y"=0.0, "Label"="Strip\t505", "Coord On/Off"=TRUE}, {"X"=506.0, "Y"=0.0, "Label"="Strip\t506", "Coord On/Off"=TRUE}, {"X"=507.0, "Y"=0.0, "Label"="Strip\t507", "Coord On/Off"=TRUE}, {"X"=508.0, "Y"=0.0, "Label"="Strip\t508", "Coord On/Off"=TRUE}, {"X"=509.0, "Y"=0.0, "Label"="Strip\t509", "Coord On/Off"=TRUE}, {"X"=510.0, "Y"=0.0, "Label"="Strip\t510", "Coord On/Off"=TRUE}, {"X"=511.0, "Y"=0.0, "Label"="Strip\t511", "Coord On/Off"=TRUE}, {"X"=512.0, "Y"=0.0, "Label"="Strip\t512", "Coord On/Off"=TRUE}, {"X"=513.0, "Y"=0.0, "Label"="Strip\t513", "Coord On/Off"=TRUE}, {"X"=514.0, "Y"=0.0, "Label"="Strip\t514", "Coord On/Off"=TRUE}, {"X"=515.0, "Y"=0.0, "Label"="Strip\t515", "Coord On/Off"=TRUE}, {"X"=516.0, "Y"=0.0, "Label"="Strip\t516", "Coord On/Off"=TRUE}, {"X"=517.0, "Y"=0.0, "Label"="Strip\t517", "Coord On/Off"=TRUE}, {"X"=518.0, "Y"=0.0, "Label"="Strip\t518", "Coord On/Off"=TRUE}, {"X"=519.0, "Y"=0.0, "Label"="Strip\t519", "Coord On/Off"=TRUE}, {"X"=520.0, "Y"=0.0, "Label"="Strip\t520", "Coord On/Off"=TRUE}, {"X"=521.0, "Y"=0.0, "Label"="Strip\t521", "Coord On/Off"=TRUE}, {"X"=522.0, "Y"=0.0, "Label"="Strip\t522", "Coord On/Off"=TRUE}, {"X"=523.0, "Y"=0.0, "Label"="Strip\t523", "Coord On/Off"=TRUE}, {"X"=524.0, "Y"=0.0, "Label"="Strip\t524", "Coord On/Off"=TRUE}, {"X"=525.0, "Y"=0.0, "Label"="Strip\t525", "Coord On/Off"=TRUE}, {"X"=526.0, "Y"=0.0, "Label"="Strip\t526", "Coord On/Off"=TRUE}, {"X"=527.0, "Y"=0.0, "Label"="Strip\t527", "Coord On/Off"=TRUE}, {"X"=528.0, "Y"=0.0, "Label"="Strip\t528", "Coord On/Off"=TRUE}, {"X"=529.0, "Y"=0.0, "Label"="Strip\t529", "Coord On/Off"=TRUE}, {"X"=530.0, "Y"=0.0, "Label"="Strip\t530", "Coord On/Off"=TRUE}, {"X"=531.0, "Y"=0.0, "Label"="Strip\t531", "Coord On/Off"=TRUE}, {"X"=532.0, "Y"=0.0, "Label"="Strip\t532", "Coord On/Off"=TRUE}, {"X"=533.0, "Y"=0.0, "Label"="Strip\t533", "Coord On/Off"=TRUE}, {"X"=534.0, "Y"=0.0, "Label"="Strip\t534", "Coord On/Off"=TRUE}, {"X"=535.0, "Y"=0.0, "Label"="Strip\t535", "Coord On/Off"=TRUE}, {"X"=536.0, "Y"=0.0, "Label"="Strip\t536", "Coord On/Off"=TRUE}, {"X"=537.0, "Y"=0.0, "Label"="Strip\t537", "Coord On/Off"=TRUE}, {"X"=538.0, "Y"=0.0, "Label"="Strip\t538", "Coord On/Off"=TRUE}, {"X"=539.0, "Y"=0.0, "Label"="Strip\t539", "Coord On/Off"=TRUE}, {"X"=540.0, "Y"=0.0, "Label"="Strip\t540", "Coord On/Off"=TRUE}, {"X"=541.0, "Y"=0.0, "Label"="Strip\t541", "Coord On/Off"=TRUE}, {"X"=542.0, "Y"=0.0, "Label"="Strip\t542", "Coord On/Off"=TRUE}, {"X"=543.0, "Y"=0.0, "Label"="Strip\t543", "Coord On/Off"=TRUE}, {"X"=544.0, "Y"=0.0, "Label"="Strip\t544", "Coord On/Off"=TRUE}, {"X"=545.0, "Y"=0.0, "Label"="Strip\t545", "Coord On/Off"=TRUE}, {"X"=546.0, "Y"=0.0, "Label"="Strip\t546", "Coord On/Off"=TRUE}, {"X"=547.0, "Y"=0.0, "Label"="Strip\t547", "Coord On/Off"=TRUE}, {"X"=548.0, "Y"=0.0, "Label"="Strip\t548", "Coord On/Off"=TRUE}, {"X"=549.0, "Y"=0.0, "Label"="Strip\t549", "Coord On/Off"=TRUE}, {"X"=550.0, "Y"=0.0, "Label"="Strip\t550", "Coord On/Off"=TRUE}, {"X"=551.0, "Y"=0.0, "Label"="Strip\t551", "Coord On/Off"=TRUE}, {"X"=552.0, "Y"=0.0, "Label"="Strip\t552", "Coord On/Off"=TRUE}, {"X"=553.0, "Y"=0.0, "Label"="Strip\t553", "Coord On/Off"=TRUE}, {"X"=554.0, "Y"=0.0, "Label"="Strip\t554", "Coord On/Off"=TRUE}, {"X"=555.0, "Y"=0.0, "Label"="Strip\t555", "Coord On/Off"=TRUE}, {"X"=556.0, "Y"=0.0, "Label"="Strip\t556", "Coord On/Off"=TRUE}, {"X"=557.0, "Y"=0.0, "Label"="Strip\t557", "Coord On/Off"=TRUE}, {"X"=558.0, "Y"=0.0, "Label"="Strip\t558", "Coord On/Off"=TRUE}, {"X"=559.0, "Y"=0.0, "Label"="Strip\t559", "Coord On/Off"=TRUE}, {"X"=560.0, "Y"=0.0, "Label"="Strip\t560", "Coord On/Off"=TRUE}, {"X"=561.0, "Y"=0.0, "Label"="Strip\t561", "Coord On/Off"=TRUE}, {"X"=562.0, "Y"=0.0, "Label"="Strip\t562", "Coord On/Off"=TRUE}, {"X"=563.0, "Y"=0.0, "Label"="Strip\t563", "Coord On/Off"=TRUE}, {"X"=564.0, "Y"=0.0, "Label"="Strip\t564", "Coord On/Off"=TRUE}, {"X"=565.0, "Y"=0.0, "Label"="Strip\t565", "Coord On/Off"=TRUE}, {"X"=566.0, "Y"=0.0, "Label"="Strip\t566", "Coord On/Off"=TRUE}, {"X"=567.0, "Y"=0.0, "Label"="Strip\t567", "Coord On/Off"=TRUE}, {"X"=568.0, "Y"=0.0, "Label"="Strip\t568", "Coord On/Off"=TRUE}, {"X"=569.0, "Y"=0.0, "Label"="Strip\t569", "Coord On/Off"=TRUE}, {"X"=570.0, "Y"=0.0, "Label"="Strip\t570", "Coord On/Off"=TRUE}, {"X"=571.0, "Y"=0.0, "Label"="Strip\t571", "Coord On/Off"=TRUE}, {"X"=572.0, "Y"=0.0, "Label"="Strip\t572", "Coord On/Off"=TRUE}, {"X"=573.0, "Y"=0.0, "Label"="Strip\t573", "Coord On/Off"=TRUE}, {"X"=574.0, "Y"=0.0, "Label"="Strip\t574", "Coord On/Off"=TRUE}, {"X"=575.0, "Y"=0.0, "Label"="Strip\t575", "Coord On/Off"=TRUE}, {"X"=576.0, "Y"=0.0, "Label"="Strip\t576", "Coord On/Off"=TRUE}, {"X"=577.0, "Y"=0.0, "Label"="Strip\t577", "Coord On/Off"=TRUE}, {"X"=578.0, "Y"=0.0, "Label"="Strip\t578", "Coord On/Off"=TRUE}, {"X"=579.0, "Y"=0.0, "Label"="Strip\t579", "Coord On/Off"=TRUE}, {"X"=580.0, "Y"=0.0, "Label"="Strip\t580", "Coord On/Off"=TRUE}, {"X"=581.0, "Y"=0.0, "Label"="Strip\t581", "Coord On/Off"=TRUE}, {"X"=582.0, "Y"=0.0, "Label"="Strip\t582", "Coord On/Off"=TRUE}, {"X"=583.0, "Y"=0.0, "Label"="Strip\t583", "Coord On/Off"=TRUE}, {"X"=584.0, "Y"=0.0, "Label"="Strip\t584", "Coord On/Off"=TRUE}, {"X"=585.0, "Y"=0.0, "Label"="Strip\t585", "Coord On/Off"=TRUE}, {"X"=586.0, "Y"=0.0, "Label"="Strip\t586", "Coord On/Off"=TRUE}, {"X"=587.0, "Y"=0.0, "Label"="Strip\t587", "Coord On/Off"=TRUE}, {"X"=588.0, "Y"=0.0, "Label"="Strip\t588", "Coord On/Off"=TRUE}, {"X"=589.0, "Y"=0.0, "Label"="Strip\t589", "Coord On/Off"=TRUE}, {"X"=590.0, "Y"=0.0, "Label"="Strip\t590", "Coord On/Off"=TRUE}, {"X"=591.0, "Y"=0.0, "Label"="Strip\t591", "Coord On/Off"=TRUE}, {"X"=592.0, "Y"=0.0, "Label"="Strip\t592", "Coord On/Off"=TRUE}, {"X"=593.0, "Y"=0.0, "Label"="Strip\t593", "Coord On/Off"=TRUE}, {"X"=594.0, "Y"=0.0, "Label"="Strip\t594", "Coord On/Off"=TRUE}, {"X"=595.0, "Y"=0.0, "Label"="Strip\t595", "Coord On/Off"=TRUE}, {"X"=596.0, "Y"=0.0, "Label"="Strip\t596", "Coord On/Off"=TRUE}, {"X"=597.0, "Y"=0.0, "Label"="Strip\t597", "Coord On/Off"=TRUE}, {"X"=598.0, "Y"=0.0, "Label"="Strip\t598", "Coord On/Off"=TRUE}, {"X"=599.0, "Y"=0.0, "Label"="Strip\t599", "Coord On/Off"=TRUE}, {"X"=600.0, "Y"=0.0, "Label"="Strip\t600", "Coord On/Off"=TRUE}, {"X"=601.0, "Y"=0.0, "Label"="Strip\t601", "Coord On/Off"=TRUE}, {"X"=602.0, "Y"=0.0, "Label"="Strip\t602", "Coord On/Off"=TRUE}, {"X"=603.0, "Y"=0.0, "Label"="Strip\t603", "Coord On/Off"=TRUE}, {"X"=604.0, "Y"=0.0, "Label"="Strip\t604", "Coord On/Off"=TRUE}, {"X"=605.0, "Y"=0.0, "Label"="Strip\t605", "Coord On/Off"=TRUE}, {"X"=606.0, "Y"=0.0, "Label"="Strip\t606", "Coord On/Off"=TRUE}, {"X"=607.0, "Y"=0.0, "Label"="Strip\t607", "Coord On/Off"=TRUE}, {"X"=608.0, "Y"=0.0, "Label"="Strip\t608", "Coord On/Off"=TRUE}, {"X"=609.0, "Y"=0.0, "Label"="Strip\t609", "Coord On/Off"=TRUE}, {"X"=610.0, "Y"=0.0, "Label"="Strip\t610", "Coord On/Off"=TRUE}, {"X"=611.0, "Y"=0.0, "Label"="Strip\t611", "Coord On/Off"=TRUE}, {"X"=612.0, "Y"=0.0, "Label"="Strip\t612", "Coord On/Off"=TRUE}, {"X"=613.0, "Y"=0.0, "Label"="Strip\t613", "Coord On/Off"=TRUE}, {"X"=614.0, "Y"=0.0, "Label"="Strip\t614", "Coord On/Off"=TRUE}, {"X"=615.0, "Y"=0.0, "Label"="Strip\t615", "Coord On/Off"=TRUE}, {"X"=616.0, "Y"=0.0, "Label"="Strip\t
